vi "GrobaLimitVoltage.vi"() -> ()   [LabVIEW 2016]
panel:
  in  "Debug":bool
  in  "Probe SN":string
  in  "Monitor Reset":bool
  in  "Reset Monitor":string
  out "Boolean":bool
  out "Output Limit Voltage":i16
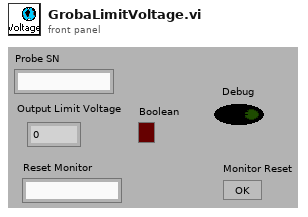
[diagram p1: front panel]
diagram:
